vi "Start (App INI).vi"(8 "error in (no error)":errorcluster, 10 "INI Path (Default)":path) -> (0 "error out":errorcluster, 2 "MessageQ":refnum<class "MessageQ.lvclass">)   [LabVIEW 2020, in "Volatus.lvlib" / "Volatus Core.lvclass"]
uses:
  Volatus Core.lvclass
  MessageQ/MessageQ.lvclass
  C:/dev/lv20CE/relink/lv-volatus/Volatus/Module/Module.lvclass
  VolatusAPI/VolatusAPI.lvclass
  VolatusConfig/VolatusConfigElement/VolatusConfigElement.lvclass
  Volatus Core.lvclass/Volatus Core.ctl
  Module/Module.lvclass
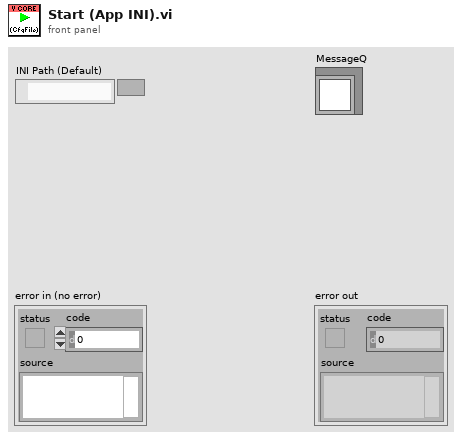
[diagram p1: front panel]
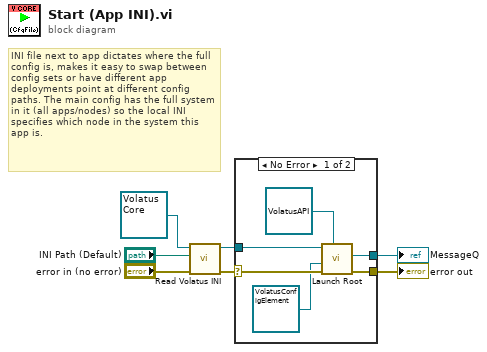
[diagram p0: block diagram]
diagram:
  # "INI file next to app dictates where the full config is, makes it easy to swap between config sets or have different app deployments point at different config paths. The main config has the full system in it (all apps/nodes) so the local INI specifies which node in the system this app is."
  n1 = call "Read Volatus INI.vi"("error in (no error)"="error in (no error)", "INI Path (Default)"="INI Path (Default)", "Volatus Core in"=refnum<class "Volatus Core.lvclass"> refnum) -> ("error out"=w1:errorcluster, "Volatus Core out"=w2:refnum<class "Volatus Core.lvclass">)  [unwired: 7 in]
  n2 = case shown="No Error" w1 {
    selector: w1 -> [w13 w14]
    tunnel: [w12 w14] -> w4
    tunnel: [w11 _] -> w5
    tunnel: w2 -> [w10 _]
    frame No Error {
      n3 = call "Launch Root.vi"("VolatusAPI"=refnum<class "VolatusAPI.lvclass"> refnum, "error in (no error)"=w13, "Config Element"=refnum<class "VolatusConfigElement.lvclass"> refnum, "Module in"=w10) -> ("error out"=w12:errorcluster, "MessageQ"=w11:refnum<class "MessageQ.lvclass">)  [unwired: 6 in]
    }
    frame Error {
    }
  }
  "error out" <- w4
  "MessageQ" <- w5
